vi "Set Slewing Test Settings.vi"(10 "Slewing Test Settings":T1 {"Settling Non-Repeating Error" format="%.4g"; "Settling Repeating Error" format="%.4g"; "Settling Time (s)" format="%.4g"; "Hold Time (s)" format="%.4g"; "Ramp Time (s)" format="%.4g"; "Max Instance Force Error (N)" format="%.4g"; "Amplitude (N)" format="%.4g"}, 11 "Model in":refnum<class "Model.lvclass">) -> (3 "Model out":refnum<class "Model.lvclass">)   [LabVIEW 2016, in "Model.lvclass"]
uses:
  Model.lvclass
  Typedefs/SlewingTestSettings.ctl
  Model.lvclass/Model.ctl
  Typedefs/FAMT Typedefs.lvlib
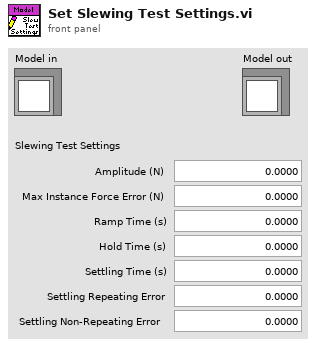
[diagram p1: front panel]
types:
  T1 = typedef "FAMT Typedefs.lvlib/SlewingTestSettings.ctl" = cluster{"Amplitude (N)":dbl, "Max Instance Force Error (N)":dbl, "Ramp Time (s)":dbl, "Hold Time (s)":dbl, "Settling Time (s)":dbl, "Settling Repeating Error":dbl, "Settling Non-Repeating Error":dbl}
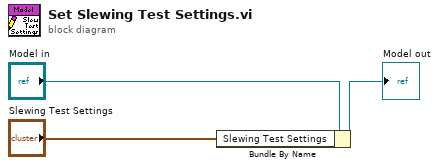
[diagram p0: block diagram]
diagram:
  n1 = Bundle By Name(cluster="Model in", "Slewing Test Settings"="Slewing Test Settings") -> (→"Model out":refnum<class "Model.lvclass">)
